vi "4296_SRX_Convert SRX Status Data.vi"(3 "Talon SRX Status in":T8) -> (1 "4296 SRX Status":T1)   [LabVIEW 2016]
uses:
  <vilib>/Rock Robotics/WPI/ThirdParty/CanMotor/TalonSRX/WPI_CANTalonSRX_GlobalStatus.ctl
  TypeDef/CLUSTER_4296_SRX_Status.ctl
  TypeDef/CLUSTER_SRX_Status Data.ctl
  TypeDef/CLUSTER_SRX_Encoder Data.ctl
  TypeDef/CLUSTER_SRX_PWM Data.ctl
  TypeDef/CLUSTER_SRX_Analog Data.ctl
  TypeDef/CLUSTER_SRX_Limit Switch Data.ctl
  TypeDef/CLUSTER_SRX_Profile Data.ctl
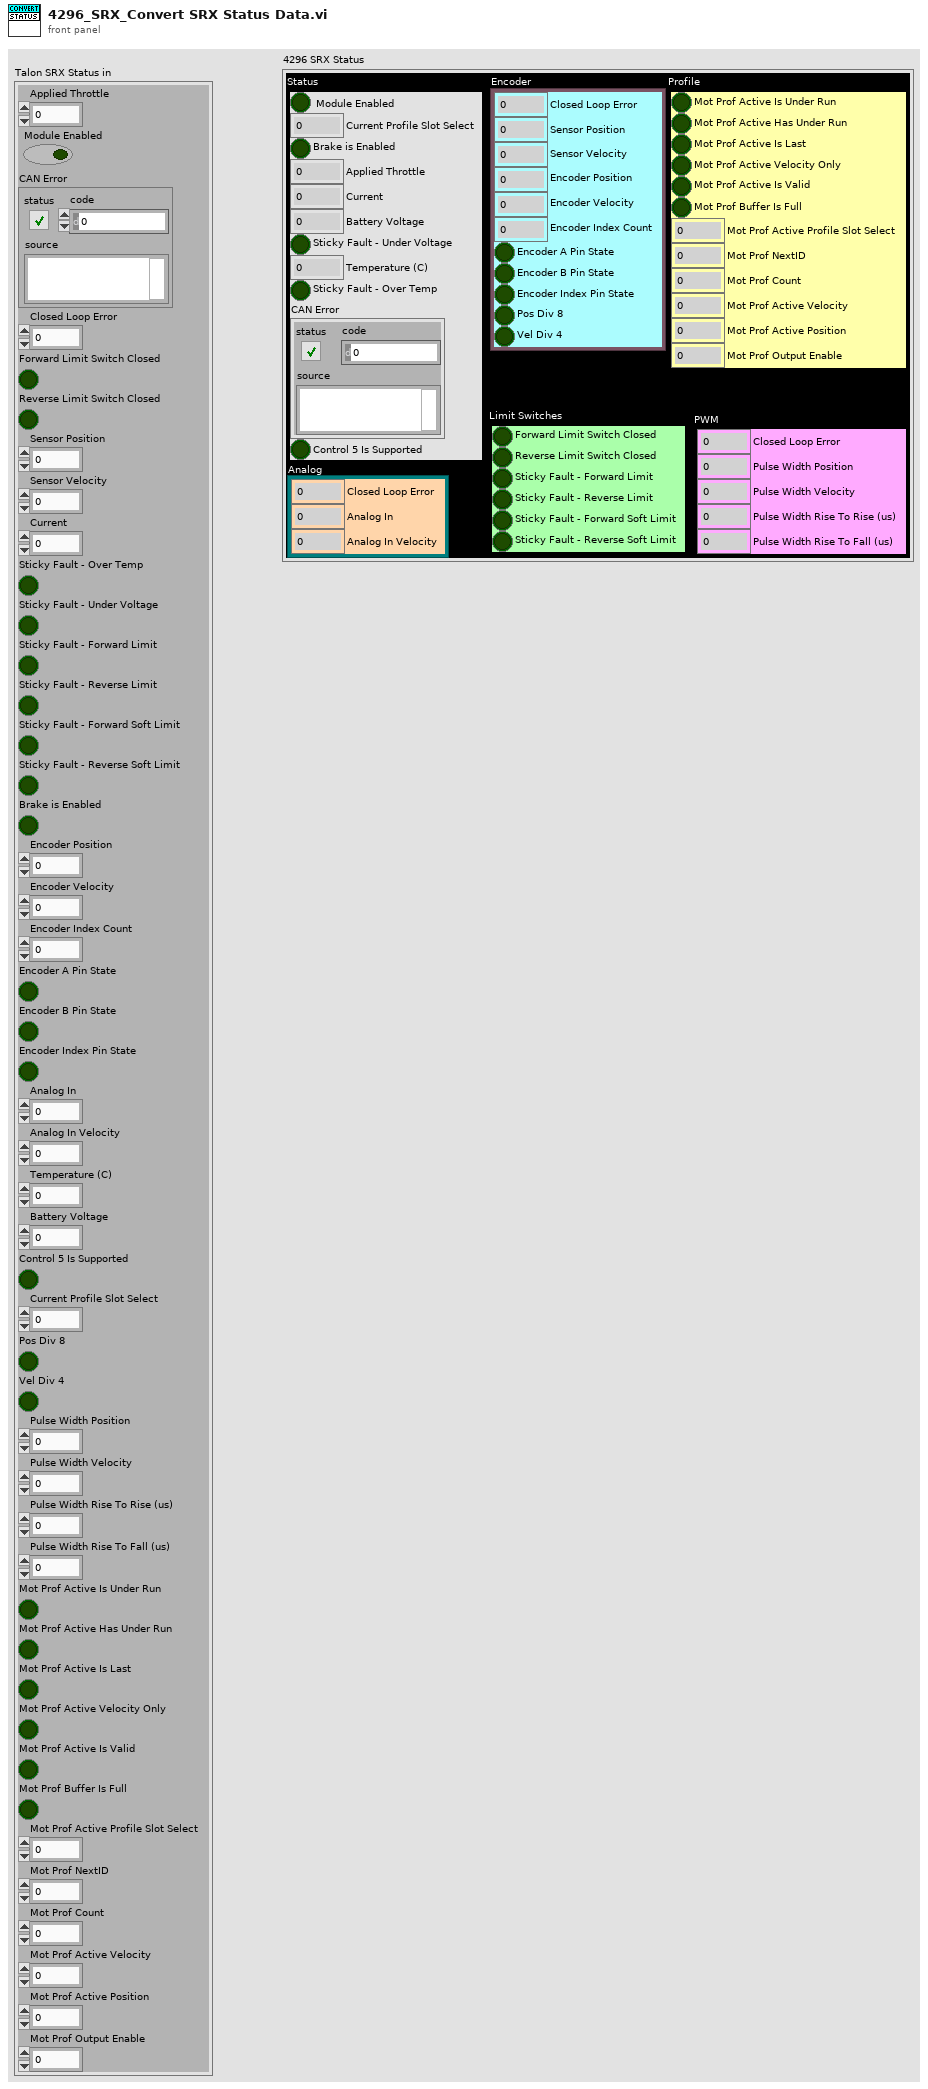
[diagram p1: front panel]
types:
  T1 = typedef "CLUSTER_4296_SRX_Status.ctl" = cluster{"Status":T2, "Encoder":T3, "PWM ":T4, "Analog":T5, "Limit Switches":T6, "Profile":T7}
  T2 = typedef "CLUSTER_SRX_Status Data.ctl" = cluster{"Module Enabled":bool, "Current Profile Slot Select":dbl, "Brake is Enabled":bool, "Applied Throttle":dbl, "Current":dbl, "Battery Voltage":dbl, "Sticky Fault - Under Voltage":bool, "Temperature (C)":dbl, "Sticky Fault - Over Temp":bool, "CAN Error":errorcluster, "Control 5 Is Supported":bool}
  T3 = typedef "CLUSTER_SRX_Encoder Data.ctl" = cluster{"Closed Loop Error":dbl, "Sensor Position":dbl, "Sensor Velocity":dbl, "Encoder Position":dbl, "Encoder Velocity":dbl, "Encoder Index Count":dbl, "Encoder A Pin State":bool, "Encoder B Pin State":bool, "Encoder Index Pin State":bool, "Pos Div 8":bool, "Vel Div 4":bool}
  T4 = typedef "CLUSTER_SRX_PWM Data.ctl" = cluster{"Closed Loop Error":dbl, "Pulse Width Position":i32, "Pulse Width Velocity":i32, "Pulse Width Rise To Rise (us)":i32, "Pulse Width Rise To Fall (us)":i32}
  T5 = typedef "CLUSTER_SRX_Analog Data.ctl" = cluster{"Closed Loop Error":dbl, "Analog In":dbl, "Analog In Velocity":dbl}
  T6 = typedef "CLUSTER_SRX_Limit Switch Data.ctl" = cluster{"Forward Limit Switch Closed":bool, "Reverse Limit Switch Closed":bool, "Sticky Fault - Forward Limit":bool, "Sticky Fault - Reverse Limit":bool, "Sticky Fault - Forward Soft Limit":bool, "Sticky Fault - Reverse Soft Limit":bool}
  T7 = typedef "CLUSTER_SRX_Profile Data.ctl" = cluster{"Mot Prof Active Is Under Run":bool, "Mot Prof Active Has Under Run":bool, "Mot Prof Active Is Last":bool, "Mot Prof Active Velocity Only":bool, "Mot Prof Active Is Valid":bool, "Mot Prof Buffer Is Full":bool, "Mot Prof Active Profile Slot Select":i32, "Mot Prof NextID":i32, "Mot Prof Count":i32, "Mot Prof Active Velocity":dbl, "Mot Prof Active Position":dbl, "Mot Prof Output Enable":i32}
  T8 = typedef "WPI_CANTalonSRX_GlobalStatus.ctl" = cluster{"Applied Throttle":dbl, "Module Enabled":bool, "CAN Error":errorcluster, "Closed Loop Error":dbl, "Forward Limit Switch Closed":bool, "Reverse Limit Switch Closed":bool, "Sensor Position":dbl, "Sensor Velocity":dbl, "Current":dbl, "Sticky Fault - Over Temp":bool, "Sticky Fault - Under Voltage":bool, "Sticky Fault - Forward Limit":bool, "Sticky Fault - Reverse Limit":bool, "Sticky Fault - Forward Soft Limit":bool, "Sticky Fault - Reverse Soft Limit":bool, "Brake is Enabled":bool, "Encoder Position":dbl, "Encoder Velocity":dbl, "Encoder Index Count":dbl, "Encoder A Pin State":bool, "Encoder B Pin State":bool, "Encoder Index Pin State":bool, "Analog In":dbl, "Analog In Velocity":dbl, "Temperature (C)":dbl, "Battery Voltage":dbl, "Control 5 Is Supported":bool, "Current Profile Slot Select":dbl, "Pos Div 8":bool, "Vel Div 4":bool, "Pulse Width Position":i32, "Pulse Width Velocity":i32, "Pulse Width Rise To Rise (us)":i32, "Pulse Width Rise To Fall (us)":i32, "Mot Prof Active Is Under Run":bool, "Mot Prof Active Has Under Run":bool, "Mot Prof Active Is Last":bool, "Mot Prof Active Velocity Only":bool, "Mot Prof Active Is Valid":bool, "Mot Prof Buffer Is Full":bool, "Mot Prof Active Profile Slot Select":i32, "Mot Prof NextID":i32, "Mot Prof Count":i32, "Mot Prof Active Velocity":dbl, "Mot Prof Active Position":dbl, "Mot Prof Output Enable":i32}
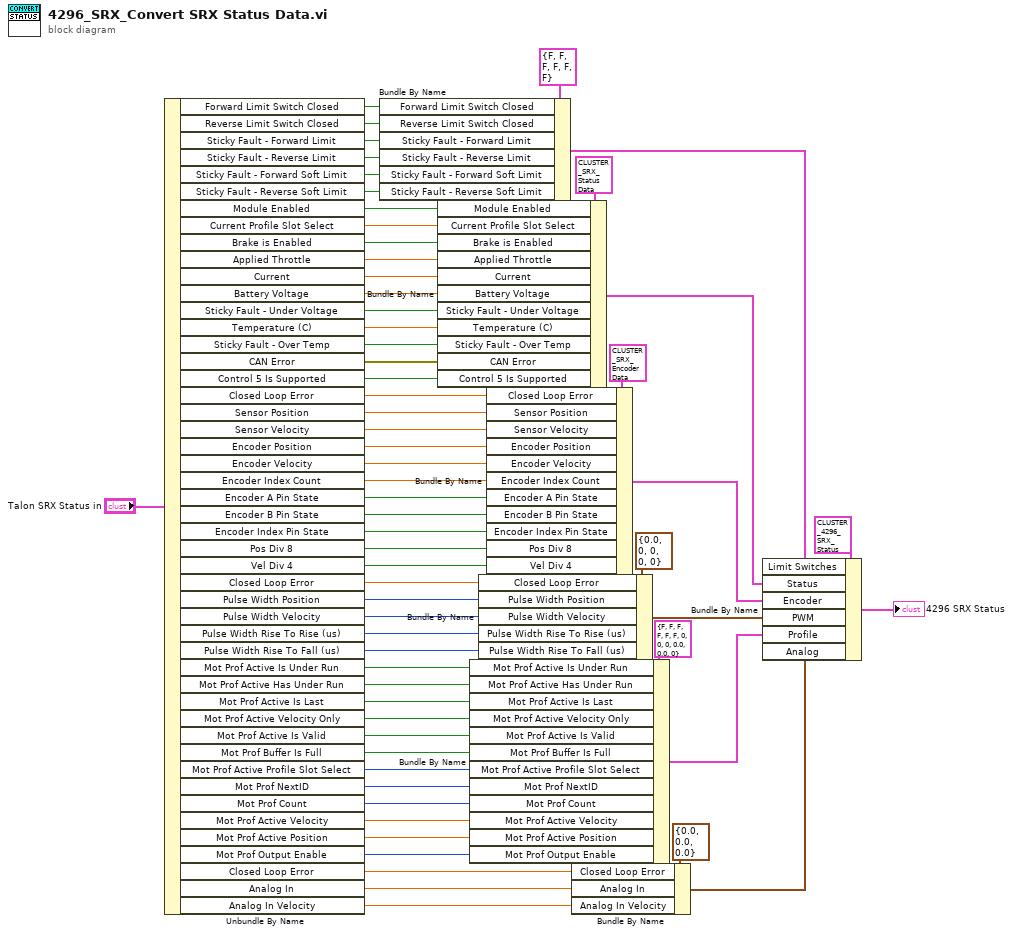
[diagram p0: block diagram]
diagram:
  n1 = Unbundle By Name("Talon SRX Status in") -> ("Forward Limit Switch Closed"=w51:bool, "Reverse Limit Switch Closed"=w52:bool, "Sticky Fault - Forward Limit"=w53:bool, "Sticky Fault - Reverse Limit"=w54:bool, "Sticky Fault - Forward Soft Limit"=w55:bool, "Sticky Fault - Reverse Soft Limit"=w56:bool, "Module Enabled"=w50:bool, "Current Profile Slot Select"=w49:dbl, "Brake is Enabled"=w48:bool, "Applied Throttle"=w47:dbl, "Current"=w46:dbl, "Battery Voltage"=w45:dbl, "Sticky Fault - Under Voltage"=w44:bool, "Temperature (C)"=w43:dbl, "Sticky Fault - Over Temp"=w42:bool, "CAN Error"=w41:errorcluster, "Control 5 Is Supported"=w40:bool, "Closed Loop Error"=w39:dbl, "Sensor Position"=w38:dbl, "Sensor Velocity"=w37:dbl, "Encoder Position"=w36:dbl, "Encoder Velocity"=w35:dbl, "Encoder Index Count"=w34:dbl, "Encoder A Pin State"=w33:bool, "Encoder B Pin State"=w32:bool, "Encoder Index Pin State"=w31:bool, "Pos Div 8"=w30:bool, "Vel Div 4"=w29:bool, "Closed Loop Error"=w28:dbl, "Pulse Width Position"=w27:i32, "Pulse Width Velocity"=w26:i32, "Pulse Width Rise To Rise (us)"=w25:i32, "Pulse Width Rise To Fall (us)"=w24:i32, "Mot Prof Active Is Under Run"=w23:bool, "Mot Prof Active Has Under Run"=w22:bool, "Mot Prof Active Is Last"=w21:bool, "Mot Prof Active Velocity Only"=w20:bool, "Mot Prof Active Is Valid"=w19:bool, "Mot Prof Buffer Is Full"=w18:bool, "Mot Prof Active Profile Slot Select"=w17:i32, "Mot Prof NextID"=w16:i32, "Mot Prof Count"=w15:i32, "Mot Prof Active Velocity"=w14:dbl, "Mot Prof Active Position"=w13:dbl, "Mot Prof Output Enable"=w12:i32, "Closed Loop Error"=w11:dbl, "Analog In"=w10:dbl, "Analog In Velocity"=w9:dbl)
  n2 = Bundle By Name(cluster=T6 {"Forward Limit Switch Closed"=FALSE, "Reverse Limit Switch Closed"=FALSE, "Sticky Fault - Forward Limit"=FALSE, "Sticky Fault - Reverse Limit"=FALSE, "Sticky Fault - Forward Soft Limit"=FALSE, "Sticky Fault - Reverse Soft Limit"=FALSE} ("Limit Switches"), "Forward Limit Switch Closed"=w51, "Reverse Limit Switch Closed"=w52, "Sticky Fault - Forward Limit"=w53, "Sticky Fault - Reverse Limit"=w54, "Sticky Fault - Forward Soft Limit"=w55, "Sticky Fault - Reverse Soft Limit"=w56) -> (w1:T6)
  n3 = Bundle By Name(cluster=T2 {"Module Enabled"=FALSE, "Current Profile Slot Select"=0.0, "Brake is Enabled"=FALSE, "Applied Throttle"=0.0, "Current"=0.0, "Battery Voltage"=0.0, "Sticky Fault - Under Voltage"=FALSE, "Temperature (C)"=0.0, "Sticky Fault - Over Temp"=FALSE, "CAN Error"={"status"=FALSE, "code"=0, "source"=""}, "Control 5 Is Supported"=FALSE} ("Status"), "Module Enabled"=w50, "Current Profile Slot Select"=w49, "Brake is Enabled"=w48, "Applied Throttle"=w47, "Current"=w46, "Battery Voltage"=w45, "Sticky Fault - Under Voltage"=w44, "Temperature (C)"=w43, "Sticky Fault - Over Temp"=w42, "CAN Error"=w41, "Control 5 Is Supported"=w40) -> (w2:T2)
  n4 = Bundle By Name(cluster=T7 {"Mot Prof Active Is Under Run"=FALSE, "Mot Prof Active Has Under Run"=FALSE, "Mot Prof Active Is Last"=FALSE, "Mot Prof Active Velocity Only"=FALSE, "Mot Prof Active Is Valid"=FALSE, "Mot Prof Buffer Is Full"=FALSE, "Mot Prof Active Profile Slot Select"=0, "Mot Prof NextID"=0, "Mot Prof Count"=0, "Mot Prof Active Velocity"=0.0, "Mot Prof Active Position"=0.0, "Mot Prof Output Enable"=0} ("Profile"), "Mot Prof Active Is Under Run"=w23, "Mot Prof Active Has Under Run"=w22, "Mot Prof Active Is Last"=w21, "Mot Prof Active Velocity Only"=w20, "Mot Prof Active Is Valid"=w19, "Mot Prof Buffer Is Full"=w18, "Mot Prof Active Profile Slot Select"=w17, "Mot Prof NextID"=w16, "Mot Prof Count"=w15, "Mot Prof Active Velocity"=w14, "Mot Prof Active Position"=w13, "Mot Prof Output Enable"=w12) -> (w4:T7)
  n5 = Bundle By Name(cluster=T4 {"Closed Loop Error"=0.0, "Pulse Width Position"=0, "Pulse Width Velocity"=0, "Pulse Width Rise To Rise (us)"=0, "Pulse Width Rise To Fall (us)"=0} ("PWM"), "Closed Loop Error"=w28, "Pulse Width Position"=w27, "Pulse Width Velocity"=w26, "Pulse Width Rise To Rise (us)"=w25, "Pulse Width Rise To Fall (us)"=w24) -> (w5:T4)
  n6 = Bundle By Name(cluster=T3 {"Closed Loop Error"=0.0, "Sensor Position"=0.0, "Sensor Velocity"=0.0, "Encoder Position"=0.0, "Encoder Velocity"=0.0, "Encoder Index Count"=0.0, "Encoder A Pin State"=FALSE, "Encoder B Pin State"=FALSE, "Encoder Index Pin State"=FALSE, "Pos Div 8"=FALSE, "Vel Div 4"=FALSE} ("Encoder"), "Closed Loop Error"=w39, "Sensor Position"=w38, "Sensor Velocity"=w37, "Encoder Position"=w36, "Encoder Velocity"=w35, "Encoder Index Count"=w34, "Encoder A Pin State"=w33, "Encoder B Pin State"=w32, "Encoder Index Pin State"=w31, "Pos Div 8"=w30, "Vel Div 4"=w29) -> (w3:T3)
  n7 = Bundle By Name(cluster=T5 {"Closed Loop Error"=0.0, "Analog In"=0.0, "Analog In Velocity"=0.0} ("Analog"), "Closed Loop Error"=w11, "Analog In"=w10, "Analog In Velocity"=w9) -> (w6:T5)
  n8 = Bundle By Name(cluster=T1 {"Status"={"Module Enabled"=FALSE, "Current Profile Slot Select"=0.0, "Brake is Enabled"=FALSE, "Applied Throttle"=0.0, "Current"=0.0, "Battery Voltage"=0.0, "Sticky Fault - Under Voltage"=FALSE, "Temperature (C)"=0.0, "Sticky Fault - Over Temp"=FALSE, "CAN Error"={"status"=FALSE, "code"=0, "source"=""}, "Control 5 Is Supported"=FALSE}, "Encoder"={"Closed Loop Error"=0.0, "Sensor Position"=0.0, "Sensor Velocity"=0.0, "Encoder Position"=0.0, "Encoder Velocity"=0.0, "Encoder Index Count"=0.0, "Encoder A Pin State"=FALSE, "Encoder B Pin State"=FALSE, "Encoder Index Pin State"=FALSE, "Pos Div 8"=FALSE, "Vel Div 4"=FALSE}, "PWM "={"Closed Loop Error"=0.0, "Pulse Width Position"=0, "Pulse Width Velocity"=0, "Pulse Width Rise To Rise (us)"=0, "Pulse Width Rise To Fall (us)"=0}, "Analog"={"Closed Loop Error"=0.0, "Analog In"=0.0, "Analog In Velocity"=0.0}, "Limit Switches"={"Forward Limit Switch Closed"=FALSE, "Reverse Limit Switch Closed"=FALSE, "Sticky Fault - Forward Limit"=FALSE, "Sticky Fault - Reverse Limit"=FALSE, "Sticky Fault - Forward Soft Limit"=FALSE, "Sticky Fault - Reverse Soft Limit"=FALSE}, "Profile"={"Mot Prof Active Is Under Run"=FALSE, "Mot Prof Active Has Under Run"=FALSE, "Mot Prof Active Is Last"=FALSE, "Mot Prof Active Velocity Only"=FALSE, "Mot Prof Active Is Valid"=FALSE, "Mot Prof Buffer Is Full"=FALSE, "Mot Prof Active Profile Slot Select"=0, "Mot Prof NextID"=0, "Mot Prof Count"=0, "Mot Prof Active Velocity"=0.0, "Mot Prof Active Position"=0.0, "Mot Prof Output Enable"=0}} ("4296 SRX Status"), "Limit Switches"=w1, "Status"=w2, "Encoder"=w3, "PWM"=w5, "Profile"=w4, "Analog"=w6) -> (→"4296 SRX Status":T1)
